vi "Customize_VI_Window.vi"() -> ()   [LabVIEW 2016]
doc: "This VI demonstrates VI Server methods and properties: Show Menu Bar, Show Title Bar, VI Transparency, and Centering the VI."
panel:
  in  "Center":bool
  in  "stop":bool
  in  "Make VI Transparent?":bool
  in  "Show Title Bar?":bool
  in  "Show Menu Bar?":bool
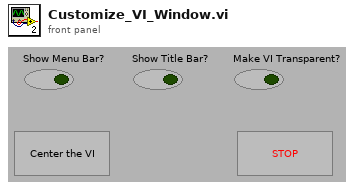
[diagram p1: front panel]
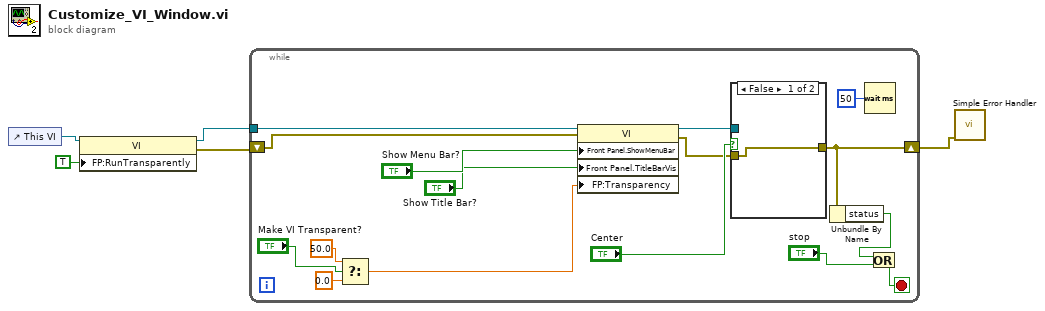
[diagram p0: block diagram]
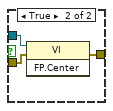
[diagram p2: hidden frame]
diagram:
  n1 = control-ref of="This VI"() -> (w5:refnum<vi>)
  n2 = property class="VI"(reference=w5, "FP:RunTransparently"=TRUE ("Front Panel Window:Run VI Transparently")) -> (reference out=w3:refnum<vi>, error out=w1:errorcluster)  [unwired: 1 in]
  n3 = while {
    tunnel: w3 -> [w16]
    shift-right: [w7] -> w2
    shift-left: w1 -> [w8]
    stop <- w11 stop-if-true
    n4 = Select(t=50.0, s="Make VI Transparent?", f=0.0) -> (s? t:f=w17:dbl)
    n5 = property class="VI"(reference=w16, error in=w8, "Front Panel.ShowMenuBar"="Show Menu Bar?", "Front Panel.TitleBarVis"="Show Title Bar?", "FP:Transparency"=w17) -> (reference out=w14:refnum<vi>, error out=w13:errorcluster)
    n6 = case shown="False" "Center" {
      tunnel: w14 -> [_ w25]
      tunnel: w13 -> [w22 w24]
      tunnel: [w22 w23] -> w7
      frame False {
      }
      frame True {
        n7 = invoke class="VI" method="FP.Center"(reference=w25, error in=w24) -> (error out=w23:errorcluster)  [unwired: 1 in, 2 out]
      }
    }
    n8 = Unbundle By Name(w7) -> ("status"=w6:bool)
    n9 = Wait (ms)(milliseconds to wait=u32 50) -> ()  [unwired: 1 out]
    n10 = Or(x=w6, y="stop") -> (x .or. y?=w11:bool)
  }
  n11 = call <vilib>:"Simple Error Handler.vi"("error in (no error)"=w2) -> ()  [unwired: 4 in, 5 out]
